vi "FVI_Trajectiore_Cercle_v2.vi"(9 "Rayon y":dbl, 10 "Rayon x":dbl, 11 "dst":dbl) -> (0 "ARG":dbl(knob) scale=-180.0..180.0, 1 "ARD":dbl(knob) scale=-180.0..180.0, 2 "AVG":dbl(knob) scale=-180.0..180.0, 3 "AVD":dbl(knob) scale=-180.0..180.0)   [LabVIEW 2018]
uses:
  <vilib>/Analysis/coordinate.llb/Angle Range (Degree).ctl
  <vilib>/Analysis/coordinate.llb/Angle Units.ctl
  <vilib>/Analysis/coordinate.llb/Wrap Angle (scalar).vi
  <vilib>/Analysis/NI_AAL_Angle.lvlib
panel:
  out "output variable":dbl
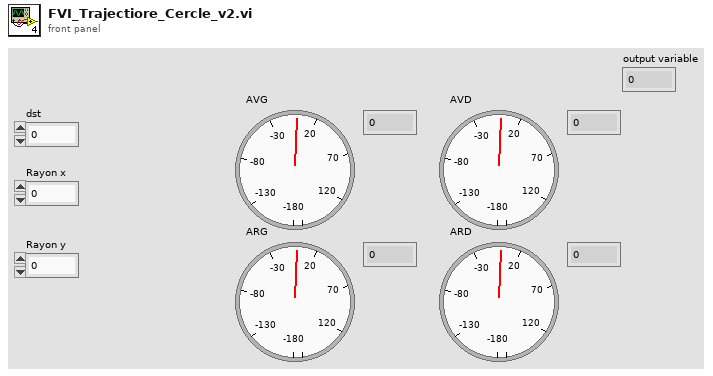
[diagram p1: front panel]
types:
  T1 = typedef "NI_AAL_Angle.lvlib/Angle Units.ctl" = i32
  T2 = typedef "NI_AAL_Angle.lvlib/Angle Range (Degree).ctl" = u16
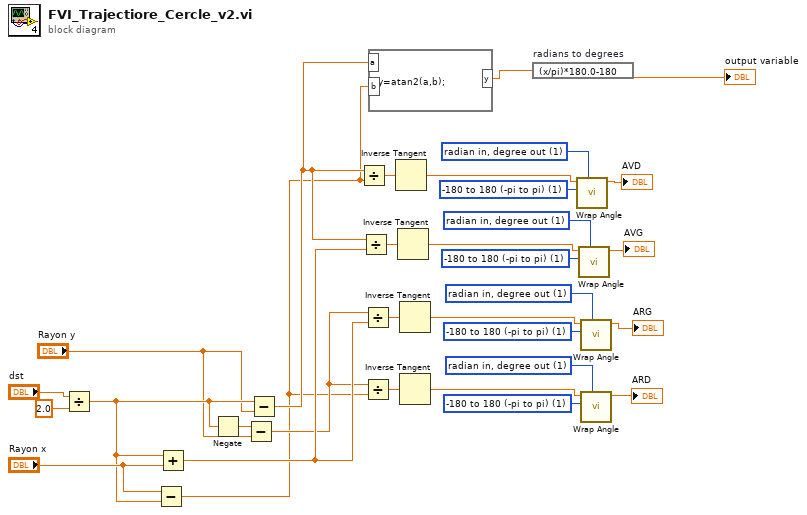
[diagram p0: block diagram]
diagram:
  w10 = T1 1 items=["radian in, radian out", "radian in, degree out", "degree in, degree out", "degree in, radian out"] ("angle units")
  w11 = T2 1 items=["none", "-180 to 180 (-pi to pi)", "0 to 360 (0 to 2pi)"] ("angle range")
  w9 = T1 1 items=["radian in, radian out", "radian in, degree out", "degree in, degree out", "degree in, radian out"] ("angle units")
  w16 = T2 1 items=["none", "-180 to 180 (-pi to pi)", "0 to 360 (0 to 2pi)"] ("angle range")
  w19 = T1 1 items=["radian in, radian out", "radian in, degree out", "degree in, degree out", "degree in, radian out"] ("angle units")
  w18 = T2 1 items=["none", "-180 to 180 (-pi to pi)", "0 to 360 (0 to 2pi)"] ("angle range")
  w25 = T1 1 items=["radian in, radian out", "radian in, degree out", "degree in, degree out", "degree in, radian out"] ("angle units")
  w26 = T2 1 items=["none", "-180 to 180 (-pi to pi)", "0 to 360 (0 to 2pi)"] ("angle range")
  n1 = Divide(x="dst", y=2.0) -> (x/y=w29:dbl)
  n2 = Subtract(x="Rayon x", y=w29) -> (x-y=w3:dbl)
  n3 = Add(x=w29, y="Rayon x") -> (x+y=w6:dbl)
  n4 = Negate(x=w29) -> (-x=w28:dbl)
  n5 = Subtract(x=w28, y="Rayon y") -> (x-y=w5:dbl)
  n6 = Subtract(x=w29, y="Rayon y") -> (x-y=w4:dbl)
  n7 = Divide(x=w4, y=w3) -> (x/y=w24:dbl)
  n8 = Divide(x=w4, y=w6) -> (x/y=w20:dbl)
  n9 = Divide(x=w5, y=w6) -> (x/y=w15:dbl)
  n10 = Divide(x=w5, y=w3) -> (x/y=w12:dbl)
  n11 = formula code="y=atan2(a,b);"("a"=w4, "b"=w3) -> ("y"=w2:dbl)
  n12 = Inverse Tangent(1:w24) -> (0:w23:dbl)
  n13 = Inverse Tangent(1:w20) -> (0:w21:dbl)
  n14 = Inverse Tangent(1:w15) -> (0:w14:dbl)
  n15 = Inverse Tangent(1:w12) -> (0:w13:dbl)
  n16 = expression code="(x/pi)*180.0-180" "radians to degrees"(w2) -> (→"output variable":dbl)
  n17 = call-poly <vilib>:"Wrap Angle.vi"("angle units"=w25, "angle range"=w26, "angle in"=w23) -> ("angle out"=→"AVD":dbl)  [unwired: 7 in, 1 out]
  n18 = call-poly <vilib>:"Wrap Angle.vi"("angle units"=w19, "angle range"=w18, "angle in"=w21) -> ("angle out"=→"AVG":dbl)  [unwired: 7 in, 1 out]
  n19 = call-poly <vilib>:"Wrap Angle.vi"("angle units"=w9, "angle range"=w16, "angle in"=w14) -> ("angle out"=→"ARG":dbl)  [unwired: 7 in, 1 out]
  n20 = call-poly <vilib>:"Wrap Angle.vi"("angle units"=w10, "angle range"=w11, "angle in"=w13) -> ("angle out"=→"ARD":dbl)  [unwired: 7 in, 1 out]
